vi "Configure Wifi.vi"(8 "Error In":errorcluster, 10 "Wifi Configuration":T1, 11 "LINX Device Config":T3) -> (0 "Error Out":errorcluster, 3 "LINX Device Config":T3)   [LabVIEW 2014, in "LMH-LINX.lvlib" / "Device.lvlib"]
uses:
  <vilib>/MakerHub/LINX/Private/Device/Device.lvlib
  <vilib>/MakerHub/LINX/Private/Device/Type Defs/LINX Device Config.ctl
  <vilib>/MakerHub/LINX/Private/Type Defs/Interface.ctl
  <vilib>/MakerHub/LINX/Private/Device/Type Defs/TCP Config.ctl
  <vilib>/MakerHub/LINX/Private/Device/Type Defs/Channels.ctl
  <vilib>/MakerHub/LINX/Private/Device/Type Defs/Wifi Config.ctl
  <vilib>/MakerHub/LINX/Private/Type Defs/WIFI Security Type.ctl
  <vilib>/MakerHub/LINX/LMH-LINX.lvlib
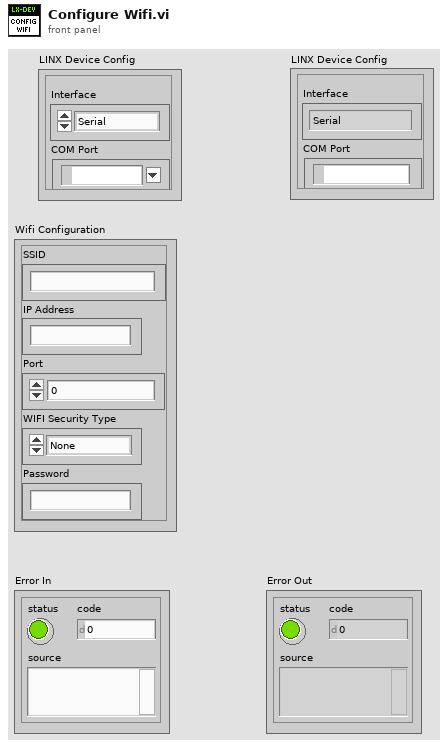
[diagram p1: front panel]
types:
  T1 = typedef "LMH-LINX.lvlib/Device.lvlib/Wifi Config.ctl" = cluster{"SSID":string, "IP Address":string, "Port":u16, "WIFI Security Type":T2, "Password":string}
  T2 = typedef "LMH-LINX.lvlib/WIFI Security Type.ctl" = enum8{"None", "WPA2 Password", "WPA2 Key", "WEP40", "WEP104"}
  T3 = typedef "LMH-LINX.lvlib/Device.lvlib/LINX Device Config.ctl" = cluster{"Interface":T4, "COM Port":refnum<visa-resource-name>, "TCP Configuration":T5, "Device Family":u8, "Device ID":u8, "Device Name":string, "TCP Ref":refnum<k5>, "Channels":T6}
  T4 = typedef "LMH-LINX.lvlib/Interface.ctl" = enum16{"Serial", "TCP"}
  T5 = typedef "LMH-LINX.lvlib/Device.lvlib/TCP Config.ctl" = cluster{"IP Address":string, "Port":u16}
  T6 = typedef "LMH-LINX.lvlib/Channels.ctl" = cluster{"DI":u8[], "DO":u8[], "AI":u8[], "AO":u8[], "PWM":u8[], "QE":u8[], "UART":u8[], "I2C 2":u8[], "SPI":u8[], "CAN":u8[], "Servo":u8[], "AI Ref (V)":dbl, "AI Resolution (Bits)":u8, "AO Ref (V)":dbl, "AO Resolution (Bits)":u8}
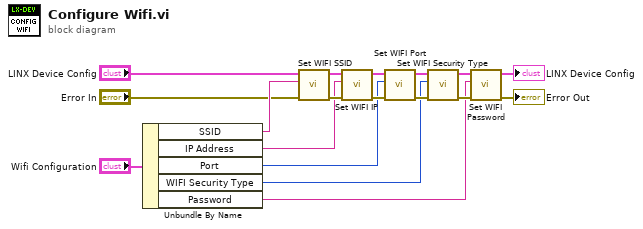
[diagram p0: block diagram]
diagram:
  n1 = Unbundle By Name("Wifi Configuration") -> ("SSID"=w9:string, "IP Address"=w8:string, "Port"=w7:u16, "WIFI Security Type"=w1:T2, "Password"=w2:string)
  n2 = call <vilib>:"Set WIFI SSID.vi"("Error In"="Error In", "SSID"=w9, "LINX Device Config"="LINX Device Config") -> ("Error Out"=w10:errorcluster, "LINX Device Config"=w13:T3)  [unwired: 7 in]
  n3 = call <vilib>:"Set WIFI IP.vi"("Error In"=w10, "IP Address"=w8, "LINX Device Config"=w13) -> ("Error Out"=w11:errorcluster, "LINX Device Config"=w12:T3)  [unwired: 7 in]
  n4 = call <vilib>:"Set WIFI Port.vi"("Error In"=w11, "Port"=w7, "LINX Device Config"=w12) -> ("Error Out"=w14:errorcluster, "LINX Device Config"=w17:T3)  [unwired: 7 in]
  n5 = call <vilib>:"Set WIFI Security Type.vi"("Error In"=w14, "WIFI Security Type"=w1, "LINX Device Config"=w17) -> ("Error Out"=w15:errorcluster, "LINX Device Config"=w16:T3)  [unwired: 7 in]
  n6 = call <vilib>:"Set WIFI Password.vi"("Error In"=w15, "Password"=w2, "LINX Device Config"=w16) -> ("Error Out"=→"Error Out":errorcluster, "LINX Device Config"=→"LINX Device Config":T3)  [unwired: 7 in]
